vi "aft_xmpl_Simulate Expected Waveform.vi"() -> (3 "Expected Waveform":dbl[](array[numeric]))   [LabVIEW 2023]
uses:
  <vilib>/Analysis/3filter.llb/FIR Filter (DBL).vi
  <vilib>/Analysis/NI_AALBase.lvlib
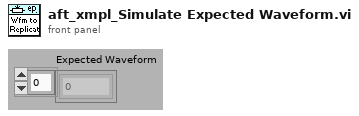
[diagram p1: front panel]
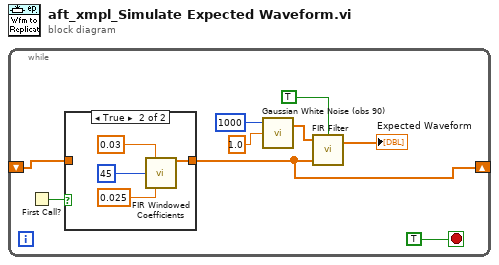
[diagram p0: block diagram]
diagram:
  n1 = while {
    shift-right: [w2] -> _
    shift-left: _ -> [w1]
    stop <- TRUE stop-if-true
    n2 = First Call?() -> (First Call?: T/F=w4:bool)
    n3 = case shown="True" w4 {
      tunnel: [w10 w11] -> w2
      tunnel: w1 -> [w10 _]
      frame False {
      }
      frame True {
        n4 = call <vilib>:"FIR Windowed Coefficients.vi"("high cutoff freq: fh"=0.03, "taps"=45, "low cutoff freq: fl"=0.025) -> ("FIR Windowed Coefficients"=w11:dbl[])  [unwired: 5 in, 7 out]
      }
    }
    n5 = call <vilib>:"Gaussian White Noise (obs 90).vi"("standard deviation"=1.0 ("amplitude"), "samples"=1000) -> ("Gaussian noise pattern"=w6:dbl[])  [unwired: 1 in, 1 out]
    n6 = call-poly <vilib>:"FIR Filter.vi"("init/cont (init:F)"=TRUE, "FIR Coefficients"=w2, "X"=w6) -> ("Filtered X"=→"Expected Waveform":dbl[])  [unwired: 1 in, 1 out]
  }
